vi "16_SynchronizedMeasurements.vi"(8 "error in (no error)":errorcluster) -> (0 "error out":errorcluster)   [LabVIEW 2014]
uses:
  SwabianInstruments.TimeTagger
panel:
  out "FileWriter files":string[](array[string])
  out "First timestamp\ndifference":dbl[unit] format="%#.2g"
  out "Time-tag display":T1(graph)
  out "all time-tags\nidentical?":bool
  in  "Start synchronously if available":bool=TRUE
  in  "Use SynchronizedMeasurements":bool=TRUE
  # "This example demonstrates the SynchronizedMeasurements class. The time-tag stream is investigated by a TimeTagStream measurement and simultaneously dumped by a FileWriter measurement. Afterward, the resulting time-tag streams are compared.\n\nSynchronizedMeasurements ensures that both sub-measurements, TimeTagStream and FileWriter, process the very same set of time-tags. It can be activated/deactivated by the \"Use SynchronizedMeasurements\" control. Even with SynchronizedMeasurements, the sub-measurements can be controlled individually (use \"start synchronously if available\" to toggle behavior.\n\nSynchronizedMeasurements has an important impact on the FileWriter: It deactivates the autostart behavior. Without SynchronizedMeasurements, autostart + startFor results in two FileWriter data files, dump.1.ttbin and dump.2.ttbin."
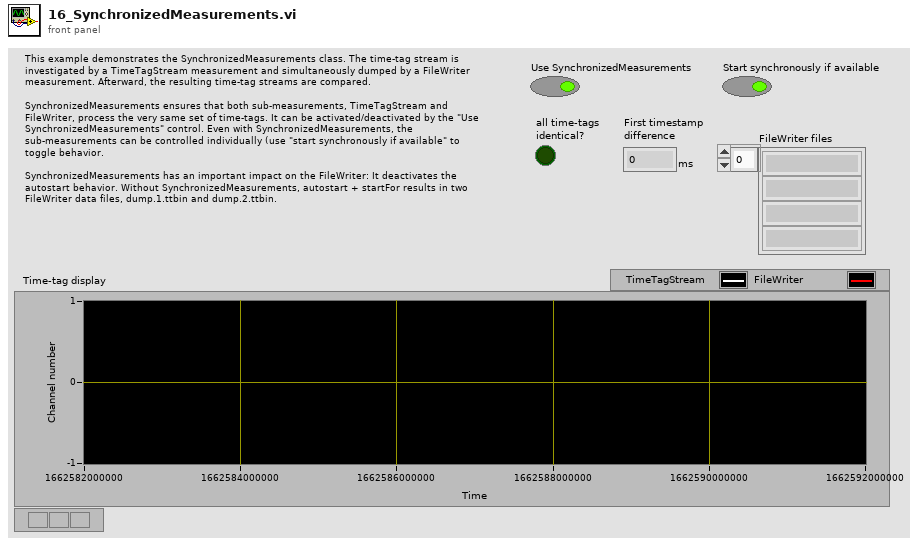
[diagram p1: front panel]
types:
  T1 = cluster{"getTimestamps":i64[], "getChannels":i32[]}[]
  T2 = cluster{"getTimestamps":i64[], "getChannels":i32[]}
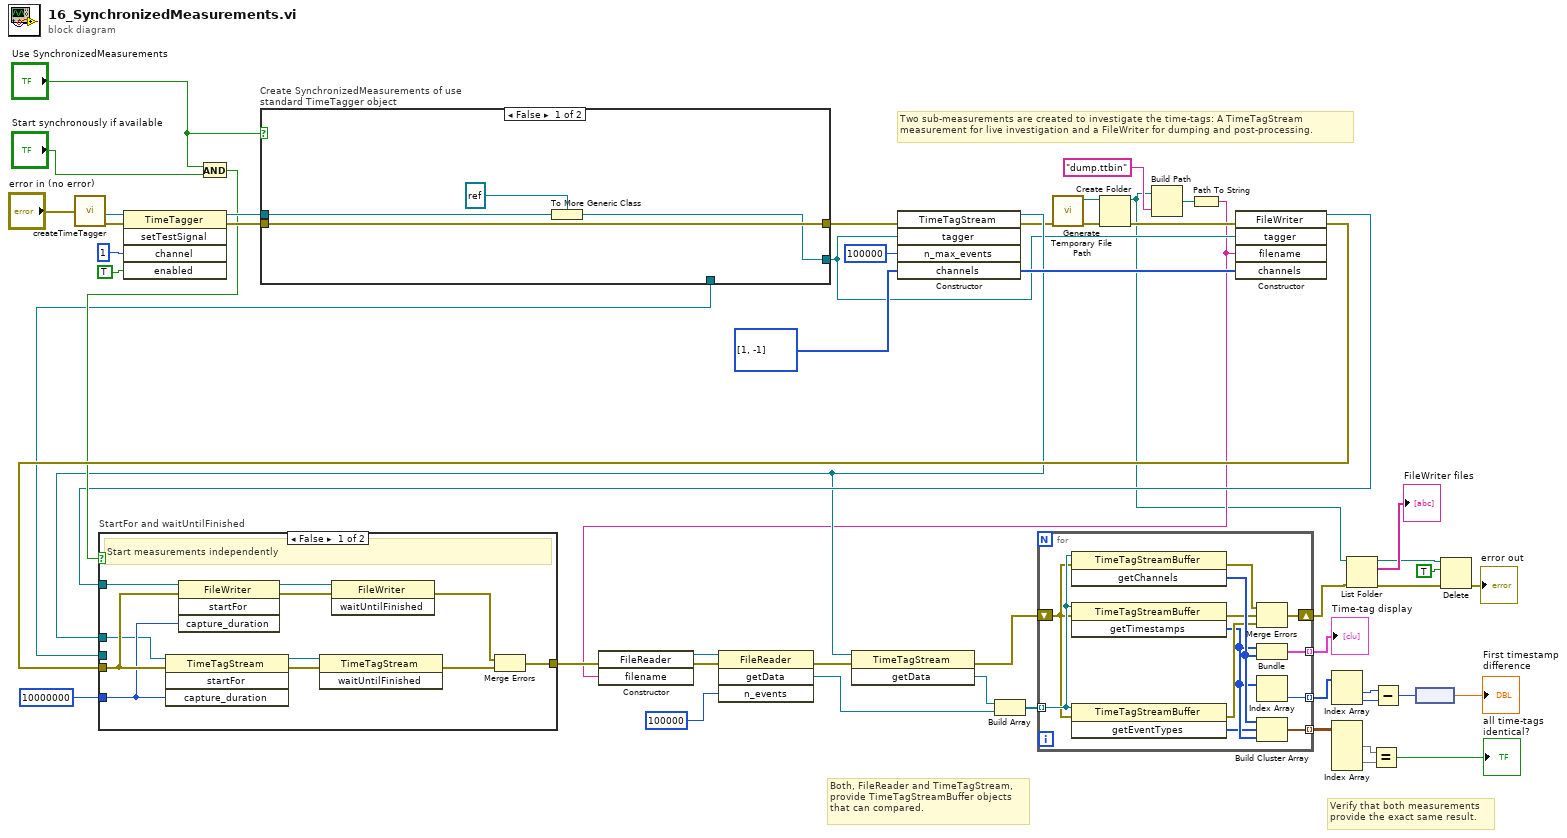
[diagram p0: block diagram]
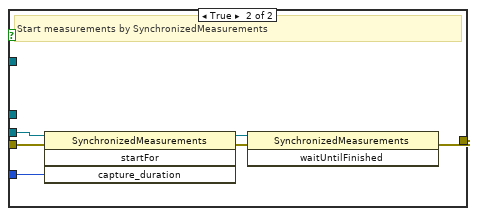
[diagram p2: hidden frame]
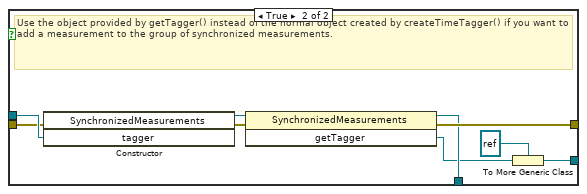
[diagram p3: hidden frame]
diagram:
  # "Both, FileReader and TimeTagStream,\nprovide TimeTagStreamBuffer objects\nthat can compared."
  # "Verify that both measurements\nprovide the exact same result."
  # "Two sub-measurements are created to investigate the time-tags: A TimeTagStream\nmeasurement for live investigation and a FileWriter for dumping and post-processing."
  n1 = call "createTimeTagger.vi"("error in (no error)"="error in (no error)") -> ("error out"=w47:errorcluster, "TimeTagger ref out"=w48:refnum<k24>)  [unwired: 9 in]
  n2 = invoke class="TimeTagger" method="setTestSignal"(reference=w48, error in=w47, "channel"=1, "enabled"=TRUE) -> (reference out=w51:refnum<k24>, error out=w50:errorcluster)  [unwired: 1 in, 3 out]
  n3 = And(x="Use SynchronizedMeasurements", y="Start synchronously if available") -> (x .and. y?=w45:bool)
  n4 = case "Create SynchronizedMeasurements of use standard TimeTagger object" shown="False" "Use SynchronizedMeasurements" {
    tunnel: [w54 w58] -> w16
    tunnel: [w57 w64] -> w52
    tunnel: w51 -> [w55 w63]
    tunnel: w50 -> [w57 w62]
    tunnel: [_ w61] -> w24
    frame False {
      n5 = To More Generic Class(target class=refnum<k24> refnum, reference=w55) -> (generic class reference=w54:refnum<k24>)
    }
    frame True {
      # "Use the object provided by getTagger() instead of the normal object created by createTimeTagger() if you want to add a measurement to the group of synchronized measurements."
      n6 = constructor class="SynchronizedMeasurements"(error in=w62, "tagger"=w63) -> (reference out=w66:refnum<k24>, error out=w65:errorcluster)  [unwired: 2 in, 2 out]
      n7 = invoke class="SynchronizedMeasurements" method="getTagger"(reference=w66, error in=w65) -> (reference out=w61:refnum<k24>, error out=w64:errorcluster, "getTagger"=w60:refnum<k24>)  [unwired: 1 in]
      n8 = To More Generic Class(target class=refnum<k24> refnum, reference=w60) -> (generic class reference=w58:refnum<k24>)
    }
  }
  n9 = constructor class="TimeTagStream"(error in=w52, "tagger"=w16, "n_max_events"=u64 100000, "channels"=i32[] [1, -1]) -> (reference out=w22:refnum<k24>, error out=w7:errorcluster, "channels"=w25:i32[])  [unwired: 2 in, 3 out]
  n10 = call <vilib>:"Generate Temporary File Path.vi"("error in (no error)"=w7) -> ("error out"=w9:errorcluster, "Unique Temporary File Path"=w8:path)  [unwired: 9 in]
  n11 = Create Folder(path (use dialog)=w8, error in=w9) -> (created path=w3:path, error out=w6:errorcluster)  [unwired: 1 in, 1 out]
  n12 = Build Path(base path=w3, name or relative path="dump.ttbin") -> (appended path=w5:path)
  n13 = Path To String(path=w5) -> (string=w4:string)
  n14 = constructor class="FileWriter"(error in=w6, "tagger"=w16, "filename"=w4, "channels"=w25) -> (reference out=w43:refnum<k24>, error out=w49:errorcluster)  [unwired: 2 in, 4 out]
  n15 = case "StartFor and waitUntilFinished" shown="False" w45 {
    tunnel: w49 -> [w73 w83]
    tunnel: w24 -> [_ w82]
    tunnel: [w69 w79] -> w20
    tunnel: i64 10000000 ("capture_duration") -> [w72 w78]
    tunnel: w22 -> [w67 _]
    tunnel: w43 -> [w68 _]
    frame False {
      # "Start measurements independently"
      n16 = invoke class="TimeTagStream" method="startFor"(reference=w67, error in=w73, "capture_duration"=w72) -> (reference out=w75:refnum<k24>, error out=w74:errorcluster)  [unwired: 1 in, 2 out]
      n17 = invoke class="FileWriter" method="startFor"(reference=w68, error in=w73, "capture_duration"=w72) -> (reference out=w77:refnum<k24>, error out=w76:errorcluster)  [unwired: 1 in, 2 out]
      n18 = invoke class="TimeTagStream" method="waitUntilFinished"(reference=w75, error in=w74) -> (error out=w70:errorcluster)  [unwired: 1 in, 2 out]
      n19 = invoke class="FileWriter" method="waitUntilFinished"(reference=w77, error in=w76) -> (error out=w71:errorcluster)  [unwired: 1 in, 2 out]
      n20 = Merge Errors(w71, w70) -> (w69:errorcluster)
    }
    frame True {
      # "Start measurements by SynchronizedMeasurements"
      n21 = invoke class="SynchronizedMeasurements" method="startFor"(reference=w82, error in=w83, "capture_duration"=w78) -> (reference out=w81:refnum<k24>, error out=w80:errorcluster)  [unwired: 1 in, 2 out]
      n22 = invoke class="SynchronizedMeasurements" method="waitUntilFinished"(reference=w81, error in=w80) -> (error out=w79:errorcluster)  [unwired: 1 in, 2 out]
    }
  }
  n23 = constructor class="FileReader"(error in=w20, "filename"=w4) -> (reference out=w42:refnum<k24>, error out=w41:errorcluster)  [unwired: 2 in, 2 out]
  n24 = invoke class="FileReader" method="getData"(reference=w42, error in=w41, "n_events"=u64 100000) -> (error out=w18:errorcluster, "getData"=w33:refnum<k24>)  [unwired: 1 in, 2 out]
  n25 = invoke class="TimeTagStream" method="getData"(reference=w22, error in=w18) -> (error out=w17:errorcluster, "getData"=w40:refnum<k24>)  [unwired: 1 in, 1 out]
  n26 = Build Array(w40, w33) -> (w39:refnum<k24>[])
  n27 = for {
    tunnel: w39 -> [w95] mode=indexing
    tunnel: [w94] -> w38 mode=indexing
    tunnel: [w93] -> w34 mode=indexing
    shift-right: [w87] -> w13
    shift-left: w17 -> [w91]
    tunnel: [w85] -> w32 mode=indexing
    n28 = invoke class="TimeTagStreamBuffer" method="getChannels"(reference=w95, error in=w91) -> (error out=w88:errorcluster, "getChannels"=w92:i32[])  [unwired: 1 in, 1 out]
    n29 = invoke class="TimeTagStreamBuffer" method="getTimestamps"(reference=w95, error in=w91) -> (error out=w89:errorcluster, "getTimestamps"=w86:i64[])  [unwired: 1 in, 1 out]
    n30 = invoke class="TimeTagStreamBuffer" method="getEventTypes"(reference=w95, error in=w91) -> (error out=w90:errorcluster, "getEventTypes"=w84:u8[])  [unwired: 1 in, 1 out]
    n31 = Merge Errors(w88, w89, w90) -> (w87:errorcluster)
    n32 = Bundle("getTimestamps"=w86, "getChannels"=w92) -> (w93:T2)  [unwired: 1 in]
    n33 = Index Array(array=w86) -> (element=w85:i64)  [unwired: 1 in]
    n34 = Build Cluster Array(w92, w84, w86) -> (w94:cluster{i32, u8, i64}[])
  }
  "Time-tag display" <- w34
  n35 = Index Array(array=w32) -> (element #1=w31:i64, element #2=w30:i64)  [unwired: 2 in]
  n36 = Index Array(array=w38) -> (element #1=w37:cluster{i32, u8, i64}[], element #2=w36:cluster{i32, u8, i64}[])  [unwired: 4 in]
  n37 = List Folder(path=w3, error in=w13) -> (path out=w11:path, filenames=→"FileWriter files":string[], error out=w12:errorcluster)  [unwired: 2 in, 1 out]
  n38 = Equal?(x=w37, y=w36) -> (x = y?=→"all time-tags\nidentical?":bool)
  n39 = Subtract(x=w31, y=w30) -> (x-y=w29:i64)
  n40 = node(w29) -> (→"First timestamp\ndifference":dbl[unit])
  n41 = Delete(path (use dialog)=w11, entire hierarchy (F)=TRUE, error in=w12) -> (error out=→"error out":errorcluster)  [unwired: 2 in, 2 out]
